vi "VMI_clean_up.vi"(4 "Error In":errorcluster, 5 "Run Options":u16(ring)=1 items=["Collect Camera", "Test with Image"], 6 "Camera Session":T4, 7 "DAQ Settings":T1={"Shutters Settings"=[{"Name"="Shutter 1", "DAQ Channel/line"="Dev1/port0/line0", "Active"=FALSE}, {"Name"="Shutter 2", "DAQ Channel/line"="Dev1/port0/line1", "Active"=FALSE}], "Shutter Task"="", "Acquire Settings"=[{"Name"="Power", "DAQ Channel/line"="Dev1/ai0", "Max V"=5.0, "Min V"=-5.0, "input terminal configuration"=10106, "Active"=FALSE}, {"Name"="Pressure 1", "DAQ Channel/line"="Dev1/ai1", "Max V"=5.0, "Min V"=-5.0, "input terminal configuration"=10106, "Active"=FALSE}, {"Name"="Pressure 2", "DAQ Channel/line"="Dev1/ai2", "Max V"=5.0, "Min V"=-5.0, "input terminal configuration"=10106, "Active"=FALSE}], "AI Task"="", "Sample mode"=10178, "Number of Samples"=100, "Rate"=1000.0, "AI Name"="Acquire", "DO Name"="Shutters"} {"Sample mode" items=["Finite Samples"=10178, "Continuous Samples"=10123, "Hardware Timed Single Point"=12522]; "Acquire Settings"."input terminal configuration" items=["default"=-1, "RSE"=10083, "NRSE"=10078, "Differential"=10106, "Pseudodifferential"=12529]}) -> (0 "Error Out":errorcluster)   [LabVIEW 2015]
uses:
  <vilib>/userdefined/High Color/IMAQdx.ctl
  Type defs/DAQ_set_Ctrl.ctl
  Type defs/DAQ_Shutter_Ctrl.ctl
  Type defs/DAQ_AI_Ctrl.ctl
  <vilib>/vision/driver/NI_Vision_Acquisition_Software.lvlib
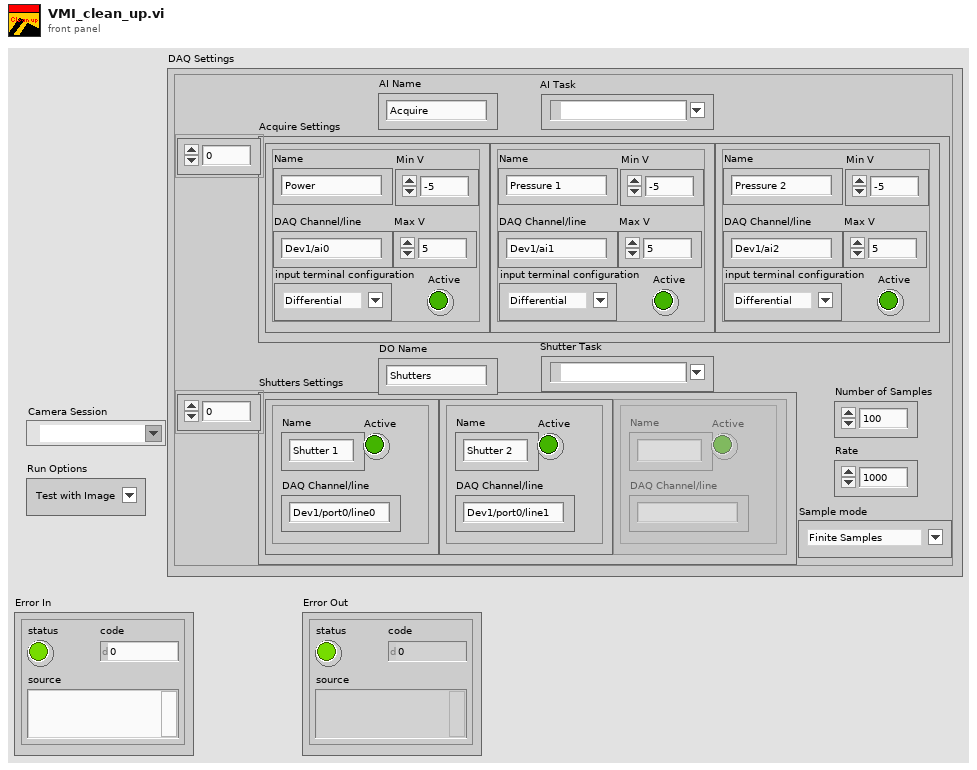
[diagram p1: front panel]
types:
  T1 = typedef "DAQ_set_Ctrl.ctl" = cluster{"Shutters Settings":T2[], "Shutter Task":refnum<k21>, "Acquire Settings":T3[], "AI Task":refnum<k21>, "Sample mode":i32, "Number of Samples":i32, "Rate":dbl, "AI Name":string, "DO Name":string}
  T2 = typedef "DAQ_Shutter_Ctrl.ctl" = cluster{"Name":string, "DAQ Channel/line":string, "Active":bool}
  T3 = typedef "DAQ_AI_Ctrl.ctl" = cluster{"Name":string, "DAQ Channel/line":string, "Max V":dbl, "Min V":dbl, "input terminal configuration":i32, "Active":bool}
  T4 = typedef "IMAQdx.ctl" = refnum<k21>
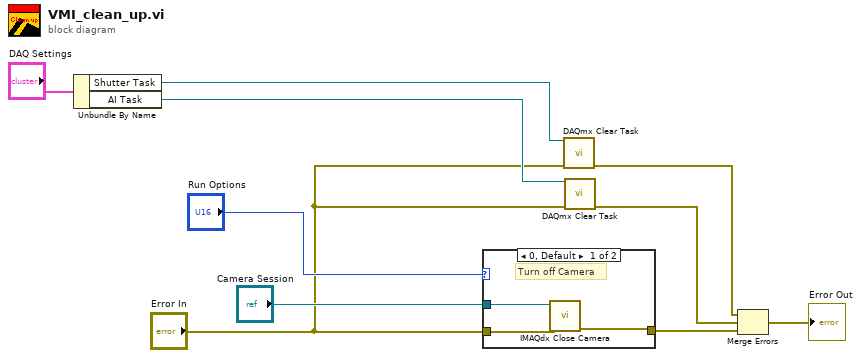
[diagram p0: block diagram]
diagram:
  n1 = Unbundle By Name("DAQ Settings") -> ("Shutter Task"=w5:refnum<k21>, "AI Task"=w4:refnum<k21>)
  n2 = case shown="0, Default" "Run Options" {
    tunnel: "Error In" -> [w12 w14]
    tunnel: "Camera Session" -> [w13 _]
    tunnel: [w11 w14] -> w10
    frame 0, Default {
      # "Turn off Camera"
      n3 = call <vilib>:"IMAQdx Close Camera.vi"("error in"=w12, "Session In"=w13) -> ("error out"=w11:errorcluster)  [unwired: 9 in]
    }
    frame 1 {
    }
  }
  n4 = call <vilib>:"DAQmx Clear Task.vi"("task in"=w5, "error in"="Error In") -> ("error out"=w2:errorcluster)  [unwired: 13 in]
  n5 = call <vilib>:"DAQmx Clear Task.vi"("task in"=w4, "error in"="Error In") -> ("error out"=w1:errorcluster)  [unwired: 13 in]
  n6 = Merge Errors(w2, w1, w10) -> (→"Error Out":errorcluster)
